vi "RightGripper.vi"(0 "error in":errorcluster, 2 "Desired Position":sgl=100.0 min=0 max=100, 3 "node":string) -> (1 "error out":errorcluster)   [LabVIEW 2015]
doc: "This will open or close the gripper to a specific position"
uses:
  ROS/Code/SubVIs/BaxterSide.ctl
panel:
  # "Gripper position is from [0.0-100.0] [close-open]"
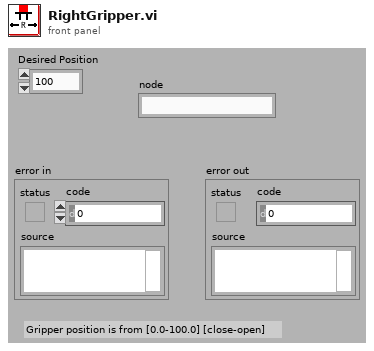
[diagram p1: front panel]
types:
  T1 = typedef "BaxterSide.ctl" = enum16{"left", "right"}
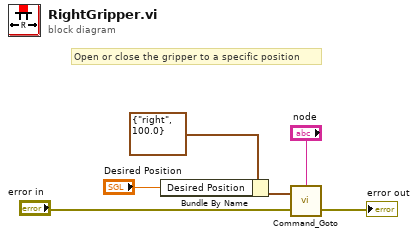
[diagram p0: block diagram]
diagram:
  # "Open or close the gripper to a specific position"
  n1 = Bundle By Name(cluster=cluster{"Side":T1, "Desired Position":sgl} {"Side"=enum."right", "Desired Position"=100.0} ("Parameters"), "Desired Position"="Desired Position") -> (w1:cluster{"Side":T1, "Desired Position":sgl})
  n2 = call "Command_Goto.vi"("error in"="error in", "Parameters"=w1, "node"="node") -> ("error out"=→"error out":errorcluster)  [unwired: 1 in]
